vi "Gesamtsystem.vi"(11 "FK":dbl) -> (3 "Beschleunigung":dbl)   [LabVIEW 2013]
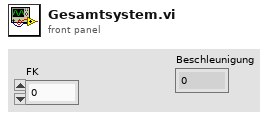
[diagram p1: front panel]
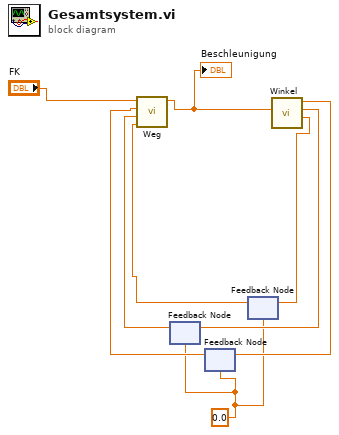
[diagram p0: block diagram]
diagram:
  w3 = 0.0
  n1 = feedback #1(w3) -> (w7:dbl)
  n2 = feedback #2(w3) -> (w6:dbl)
  n3 = feedback #3(w3) -> (w4:dbl)
  n4 = call "Weg.vi"("Fk"="FK", "p''"=w6, "p'"=w7, "Winkel"=w4) -> ("Beschleunigung"=w1:dbl)  [unwired: 3 in, 2 out]
  "Beschleunigung" <- w1
  n5 = call "Winkel.vi"("Beschleunigung"=w1) -> ("Winkel"=w5:dbl, "p'"=w8:dbl, "p''"=w9:dbl)  [unwired: 8 in]
  n6 = feedback-in #1(w8) -> ()
  n7 = feedback-in #2(w9) -> ()
  n8 = feedback-in #3(w5) -> ()
